vi "XXX_withREPLAN_PathPlanner_Cmd_Follow_Internal_Replan_Sample.vi"(4 "PassthroughTime_SEC":dbl, 5 "Extra Time Sec":dbl, 6 "Reset In":bool, 7 "ReplanningConfig":T6={"enableInitialReplanning"=TRUE, "enableDynamicReplanning"=FALSE, "dynamicReplanningTotalErrorThreshold"=1.0, "dynamicReplanningErrorSpikeThreshold"=0.25}, 8 "Position Error M":dbl, 9 "Current Pose SI":T20 {"ROTATION"."SIN" format="%13.4f"; "ROTATION"."COS" format="%13.4f"; "ROTATION"."VALUE" format="%13.4f"; "TRANSLATION"."Y" format="%14.3f"; "TRANSLATION"."X" format="%14.3f"}, 10 "CurrentChassisSpeeds":T21 {"vOmega" format="%10.3f"; "vY" format="%10.3f"; "vX" format="%10.3f"}, 11 "RePlannedPath in":T11={"Reversed"=FALSE, "RotationTargets"=[], "ConstraintZones"=[], "EventMarkers"=[], "GlobalConstraints"={"MaxVelocityMps;"=0.0, "MaxAccelerationMpsSq;"=0.0, "MaxAngularVelRadPsEc;"=0.0, "MaxAngularAccRadPSecSq"=0.0, "Exists"=FALSE, "Unlimited"=FALSE, "NominalVoltageVolts"=12.0}, "GoalEndState"={"VelocityMPS"=0.0, "Rotation"={"VALUE"=0.0, "COS"=0.0, "SIN"=0.0}}, "AllPoints"=[], "Name"="", "Waypoints"=[], "PointTowardsZones"=[], "IdealStartingState"={"VelocityMPS"=0.0, "Rotation"={"VALUE"=0.0, "COS"=0.0, "SIN"=0.0}}, "IsChoreoPath"=FALSE, "PreventFlipping"=FALSE} {"IdealStartingState"."Rotation"."SIN" format="%13.4f"; "IdealStartingState"."Rotation"."COS" format="%13.4f"; "IdealStartingState"."Rotation"."VALUE" format="%13.4f"; "PointTowardsZones"."TargetPosition"."Y" format="%14.3f"; "PointTowardsZones"."TargetPosition"."X" format="%14.3f"; "PointTowardsZones"."RotationOffset"."SIN" format="%13.4f"; "PointTowardsZones"."RotationOffset"."COS" format="%13.4f"; "PointTowardsZones"."RotationOffset"."VALUE" format="%13.4f"; "Waypoints"."nextControl"."Y" format="%14.3f"; "Waypoints"."nextControl"."X" format="%14.3f"; "Waypoints"."anchor"."Y" format="%14.3f"; "Waypoints"."anchor"."X" format="%14.3f"; "Waypoints"."prevControl"."Y" format="%14.3f"; "Waypoints"."prevControl"."X" format="%14.3f"; "AllPoints"."RotationTarget"."rotation"."SIN" format="%13.4f"; "AllPoints"."RotationTarget"."rotation"."COS" format="%13.4f"; "AllPoints"."RotationTarget"."rotation"."VALUE" format="%13.4f"; "AllPoints"."Position"."Y" format="%14.3f"; "AllPoints"."Position"."X" format="%14.3f"; "GoalEndState"."Rotation"."SIN" format="%13.4f"; "GoalEndState"."Rotation"."COS" format="%13.4f"; "GoalEndState"."Rotation"."VALUE" format="%13.4f"; "RotationTargets"."rotation"."SIN" format="%13.4f"; "RotationTargets"."rotation"."COS" format="%13.4f"; "RotationTargets"."rotation"."VALUE" format="%13.4f"}) -> (0 "Traj End Status":T5, 1 "Trajectory State":T7={"TimeSeconds"=0.0, "VelocityMPS"=0.0, "AccerationMpsSq"=0.0, "HeadingAngularVelRadPerSec"=0.0, "PositionMeters"={"X"=0.0, "Y"=0.0}, "Heading"={"VALUE"=0.0, "COS"=1.0, "SIN"=0.0}, "TargetHolonomicRotation"={"VALUE"=0.0, "COS"=1.0, "SIN"=0.0}, "CurvatureRadPerMeter"=0.0, "PathPlannerConstraints"={"MaxVelocityMps;"=0.0, "MaxAccelerationMpsSq;"=0.0, "MaxAngularVelRadPsEc;"=0.0, "MaxAngularAccRadPSecSq"=0.0, "Exists"=FALSE, "Unlimited"=FALSE, "NominalVoltageVolts"=12.0}, "DeltaPos"=0.0} {"TargetHolonomicRotation"."SIN" format="%13.4f"; "TargetHolonomicRotation"."COS" format="%13.4f"; "TargetHolonomicRotation"."VALUE" format="%13.4f"; "Heading"."SIN" format="%13.4f"; "Heading"."COS" format="%13.4f"; "Heading"."VALUE" format="%13.4f"; "PositionMeters"."Y" format="%14.3f"; "PositionMeters"."X" format="%14.3f"}, 2 "Reset Controller":bool, 3 "PathPlannerTrajectoryEvents":T1)   [LabVIEW 2019]
doc: "This is an internal function. It is not to be called by end users."
uses:
  <vilib>/Rock Robotics/WPI/ThirdParty/JAS_Junk/TrajLib/TypeDef/CHASSIS_SPEEDS.ctl
  <vilib>/Rock Robotics/WPI/ThirdParty/JAS_Junk/TrajLib/TypeDef/POSE2D.ctl
  <vilib>/Rock Robotics/WPI/ThirdParty/JAS_Junk/TrajLib/TypeDef/TRANSLATION2D.ctl
  <vilib>/Rock Robotics/WPI/ThirdParty/JAS_Junk/TrajLib/TypeDef/ROTATION2D.ctl
  PathPlannerLib24/TypeDef/PathPlannerPath.ctl
  PathPlannerLib24/TypeDef/PathPlannerRotationTarget.ctl
  PathPlannerLib24/TypeDef/PathPlannerConstraintsZone.ctl
  PathPlannerLib24/TypeDef/PathPlannerPathConstraints.ctl
  PathPlannerLib24/TypeDef/PathPlannerEventMarker.ctl
  PathPlannerLib24/TypeDef/PathPlannerCommandUtil.ctl
  PathPlannerLib24/ENum/PathPlanner_CommandUtilType_ENUM.ctl
  PathPlannerLib24/TypeDef/PathPlannerGoalEndState.ctl
  PathPlannerLib24/TypeDef/PathPlannerPathPoint.ctl
  PathPlannerLib24/TypeDef/PathPlannerWaypoint.ctl
  PathPlannerLib24/TypeDef/PathPlannerPointTowardsZone.ctl
  PathPlannerLib24/TypeDef/PathPlannerIdealStartingState.ctl
  PathPlannerLib24/TypeDef/PathPlannerTrajectoryState.ctl
  PathPlannerLib24/TypeDef/PathPlannerReplanningConfig.ctl
  PathPlannerLib24/TypeDef/PathPlannerTrajectoryEvents.ctl
  PathPlannerLib24/TypeDef/PathPlannerTrajectoryEvent.ctl
  <vilib>/Rock Robotics/WPI/ThirdParty/JAS_Junk/TrajLib/Rotation2d_GetDegrees.vi
  <vilib>/Rock Robotics/WPI/ThirdParty/JAS_Junk/TrajLib/MathUtil_InputModulus.vi
  <vilib>/Rock Robotics/WPI/ThirdParty/JAS_Junk/TrajLib/Rotation2d_CreateAngleDegrees.vi
  <vilib>/Rock Robotics/WPI/ThirdParty/JAS_Junk/TrajLib/Rotation2d_GetRadians.vi
  <vilib>/Rock Robotics/WPI/ThirdParty/JAS_Junk/TrajLib/Conv_Radians_Deg.vi
  <vilib>/Rock Robotics/WPI/ThirdParty/JAS_Junk/TrajLib/Conv_Deg_Radians.vi
  <vilib>/Rock Robotics/WPI/ThirdParty/JAS_Junk/TrajLib/Rotation2d_CreateAngle.vi
  <vilib>/Utility/semaphor.llb/Obtain Semaphore Reference.vi
  PathPlannerLib24/PathPlanner24.lvlib
  <vilib>/Rock Robotics/WPI/ThirdParty/JAS_Junk/TrajLib/Trajectory_Library.lvlib
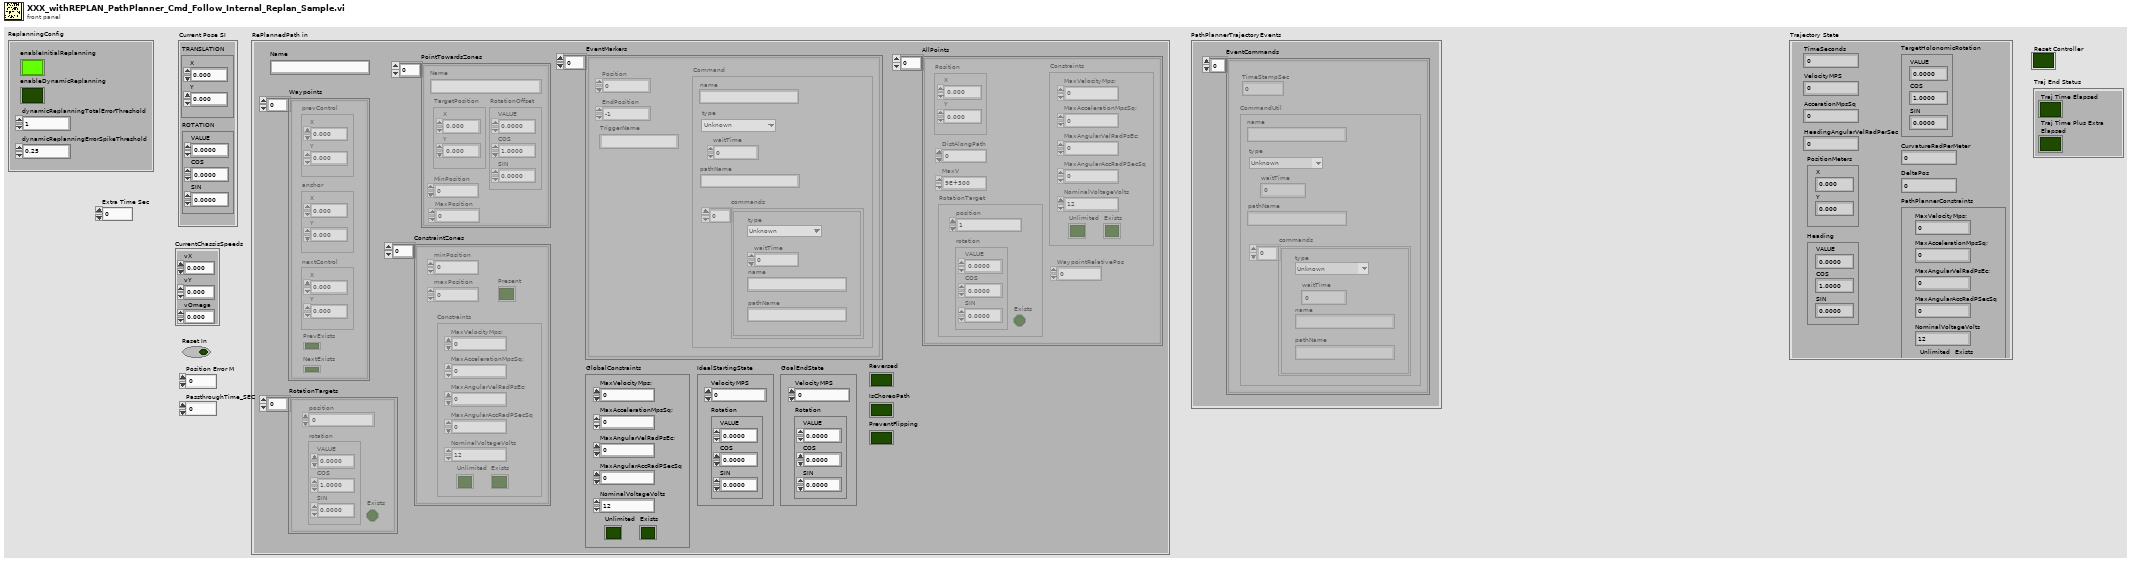
[diagram p1: front panel]
types:
  T1 = typedef "PathPlanner24.lvlib/PathPlannerTrajectoryEvents.ctl" = cluster{"EventCommands":T2[]}
  T2 = typedef "PathPlanner24.lvlib/PathPlannerTrajectoryEvent.ctl" = cluster{"TimeStampSec":dbl, "CommandUtil":T3}
  T3 = typedef "PathPlanner24.lvlib/PathPlannerCommandUtil.ctl" = cluster{"waitTime":dbl, "name":string, "pathName":string, "commands":cluster{"type":T4, "waitTime":dbl, "name":string, "pathName":string}[], "type":T4}
  T4 = typedef "PathPlanner24.lvlib/PathPlanner_CommandUtilType_ENUM.ctl" = enum16{"Unknown", "Wait", "Named", "Path", "Sequential", "Parallel", "Race", "Deadline"}
  T5 = cluster{"Traj Time Plus Extra\nElapsed":bool, "Traj Time Elapsed":bool}
  T6 = typedef "PathPlanner24.lvlib/PathPlannerReplanningConfig.ctl" = cluster{"enableInitialReplanning":bool, "enableDynamicReplanning":bool, "dynamicReplanningTotalErrorThreshold":dbl, "dynamicReplanningErrorSpikeThreshold":dbl}
  T7 = typedef "PathPlanner24.lvlib/PathPlannerTrajectoryState.ctl" = cluster{"TimeSeconds":dbl, "VelocityMPS":dbl, "AccerationMpsSq":dbl, "HeadingAngularVelRadPerSec":dbl, "PositionMeters":T8, "Heading":T9, "TargetHolonomicRotation":T9, "CurvatureRadPerMeter":dbl, "PathPlannerConstraints":T10, "DeltaPos":dbl}
  T8 = typedef "Trajectory_Library.lvlib/TRANSLATION2D.ctl" = cluster{"X":dbl, "Y":dbl}
  T9 = typedef "Trajectory_Library.lvlib/ROTATION2D.ctl" = cluster{"VALUE":dbl, "COS":dbl, "SIN":dbl}
  T10 = typedef "PathPlanner24.lvlib/PathPlannerPathConstraints.ctl" = cluster{"MaxVelocityMps;":dbl, "MaxAccelerationMpsSq;":dbl, "MaxAngularVelRadPsEc;":dbl, "MaxAngularAccRadPSecSq":dbl, "Exists":bool, "Unlimited":bool, "NominalVoltageVolts":dbl}
  T11 = typedef "PathPlanner24.lvlib/PathPlannerPath.ctl" = cluster{"Reversed":bool, "RotationTargets":T12[], "ConstraintZones":T13[], "EventMarkers":T14[], "GlobalConstraints":T10, "GoalEndState":T15, "AllPoints":T16[], "Name":string, "Waypoints":T17[], "PointTowardsZones":T18[], "IdealStartingState":T19, "IsChoreoPath":bool, "PreventFlipping":bool}
  T12 = typedef "PathPlanner24.lvlib/PathPlannerRotationTarget.ctl" = cluster{"position":dbl, "rotation":T9, "Exists":bool}
  T13 = typedef "PathPlanner24.lvlib/PathPlannerConstraintsZone.ctl" = cluster{"minPosition":dbl, "maxPosition":dbl, "Constraints":T10, "Present":bool}
  T14 = typedef "PathPlanner24.lvlib/PathPlannerEventMarker.ctl" = cluster{"Position":dbl, "Command":T3, "TriggerName":string, "EndPosition":dbl}
  T15 = typedef "PathPlanner24.lvlib/PathPlannerGoalEndState.ctl" = cluster{"VelocityMPS":dbl, "Rotation":T9}
  T16 = typedef "PathPlanner24.lvlib/PathPlannerPathPoint.ctl" = cluster{"Position":T8, "DistAlongPath":dbl, "MaxV":dbl, "Constraints":T10, "RotationTarget":T12, "WaypointRelativePos":dbl}
  T17 = typedef "PathPlanner24.lvlib/PathPlannerWaypoint.ctl" = cluster{"prevControl":T8, "anchor":T8, "nextControl":T8, "PrevExists":bool, "NextExists":bool}
  T18 = typedef "PathPlanner24.lvlib/PathPlannerPointTowardsZone.ctl" = cluster{"RotationOffset":T9, "Name":string, "TargetPosition":T8, "MinPosition":dbl, "MaxPosition":dbl}
  T19 = typedef "PathPlanner24.lvlib/PathPlannerIdealStartingState.ctl" = cluster{"VelocityMPS":dbl, "Rotation":T9}
  T20 = typedef "Trajectory_Library.lvlib/POSE2D.ctl" = cluster{"TRANSLATION":T8, "ROTATION":T9}
  T21 = typedef "Trajectory_Library.lvlib/CHASSIS_SPEEDS.ctl" = cluster{"vX":dbl, "vY":dbl, "vOmega":dbl}
  T22 = typedef "PathPlanner24.lvlib/PathPlannerTrajectory.ctl" = cluster{"States":T7[]}
  T23 = typedef "Trajectory_Library.lvlib/TIMER.ctl" = cluster{"StartTime":dbl, "Accumulated TIme":dbl, "Running":bool, "semaphore":T24}
  T24 = typedef "Semaphore RefNum" = refnum<k1>
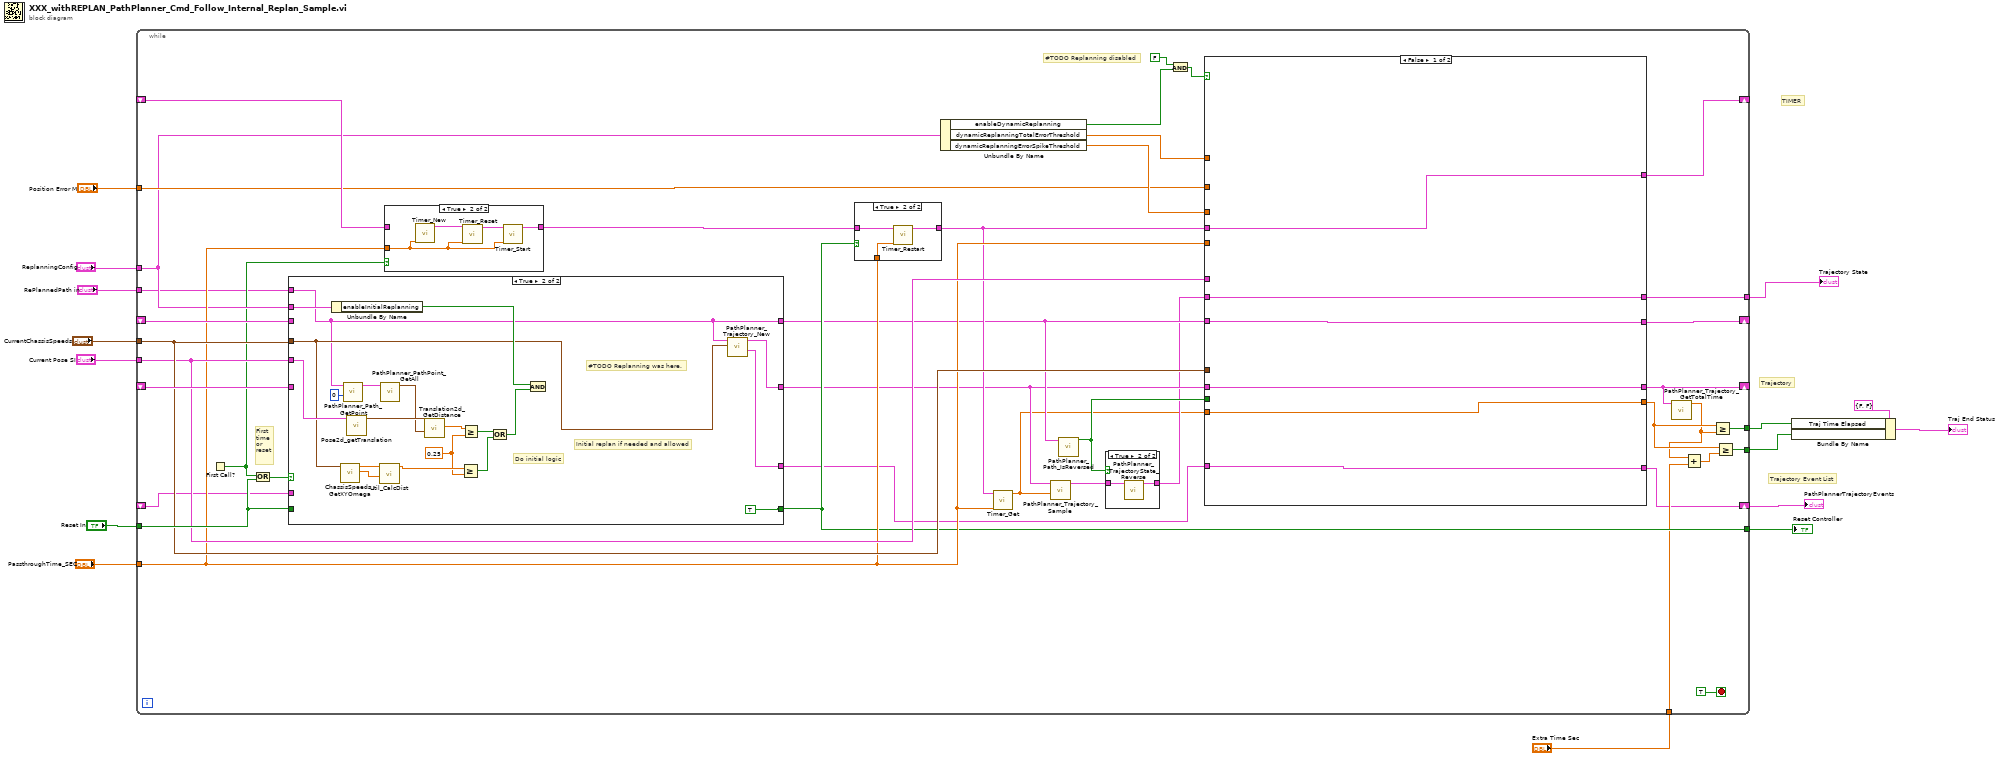
[diagram p0: block diagram]
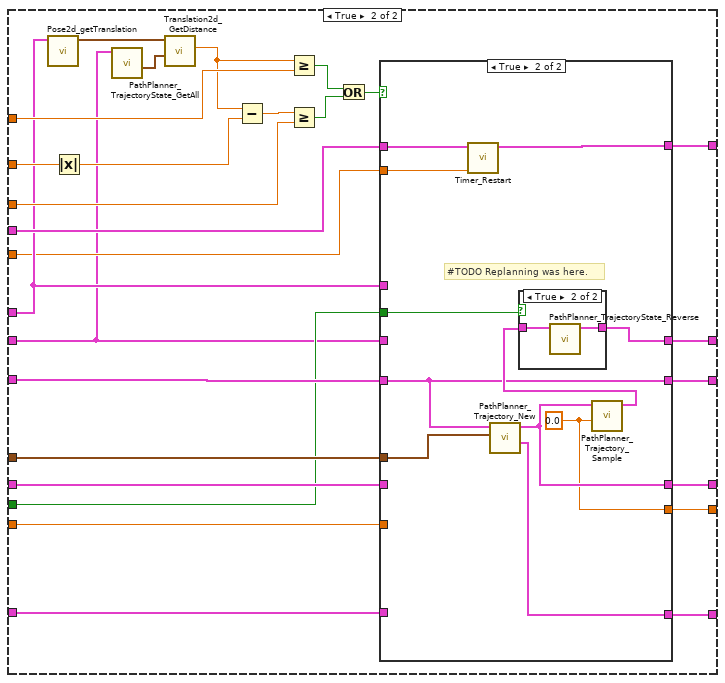
[diagram p2: hidden frame]
diagram:
  # "Trajectory Event List"
  # "TIMER"
  # "Trajectory"
  n1 = while {
    tunnel: "CurrentChassisSpeeds" -> [w50]
    tunnel: "Current Pose SI" -> [w49]
    shift-right: [w33] -> _
    shift-left: _ -> [w55]
    shift-right: [w40] -> _
    shift-left: _ -> [w54]
    tunnel: "Reset In" -> [w53]
    tunnel: [w39] -> w13
    tunnel: [w41] -> w11
    tunnel: "PassthroughTime_SEC" -> [w46]
    shift-right: [w35] -> _
    shift-left: _ -> [w47]
    tunnel: "Position Error M" -> [w38]
    tunnel: "ReplanningConfig" -> [w37]
    tunnel: [w32] -> w5
    tunnel: [w27] -> w4
    tunnel: "Extra Time Sec" -> [w26]
    shift-right: [w21] -> w1
    shift-left: _ -> [w20]
    tunnel: "RePlannedPath in" -> [w19]
    stop <- TRUE stop-if-true
    # "#TODO Replanning disabled"
    # "First\ntime\nor \nreset"
    n2 = First Call?() -> (First Call?: T/F=w34:bool)
    n3 = Or(x=w34, y=w53) -> (x .or. y?=w52:bool)
    n4 = case shown="True" w52 {
      tunnel: w54 -> [w123 _]
      tunnel: w50 -> [_ w129]
      tunnel: [w122 w128] -> w31
      tunnel: w37 -> [_ w143]
      tunnel: w49 -> [_ w130]
      tunnel: [w123 w127] -> w36
      tunnel: w55 -> [w122 _]
      tunnel: w53 -> [w124 _]
      tunnel: [w124 TRUE] -> w39
      tunnel: [w121 w125] -> w22
      tunnel: w20 -> [w121 _]
      tunnel: w19 -> [_ w127]
      frame False {
      }
      frame True {
        w132 = 0.25 ("y")
        # "#TODO Replanning was here."
        # "Initial replan if needed and allowed"
        # "Do initial logic"
        n5 = Unbundle By Name(w143) -> ("enableInitialReplanning"=w136:bool)
        n6 = call <vilib>:"ChassisSpeeds_GetXYOmega.vi"("CHASSIS"=w129) -> ("vY"=w134:dbl, "vX"=w135:dbl)  [unwired: 8 in, 1 out]
        n7 = call "PathPlanner_Path_GetPoint.vi"("Index"=0, "PathPlannerPath"=w127) -> ("Point"=w141:T16)  [unwired: 9 in]
        n8 = call <vilib>:"Pose2d_getTranslation.vi"("in POSE"=w130) -> ("outTRANSLATION"=w142:T8)  [unwired: 10 in]
        n9 = call <vilib>:"Util_CalcDist.vi"("Y"=w134, "X"=w135) -> ("DIST"=w133:dbl)  [unwired: 9 in]
        n10 = call "PathPlanner_PathPoint_GetAll.vi"("PathPlannerPoint"=w141) -> ("Position"=w140:T8)  [unwired: 5 in, 5 out]
        n11 = call <vilib>:"Translation2d_GetDistance.vi"("other Translation"=w140, "In Translation"=w142) -> ("Distance"=w139:dbl)  [unwired: 9 in]
        n12 = Greater Or Equal?(x=w133, y=w132) -> (x >= y?=w131:bool)
        n13 = Greater Or Equal?(x=w139, y=w132) -> (x >= y?=w138:bool)
        n14 = Or(x=w138, y=w131) -> (x .or. y?=w137:bool)
        n15 = And(x=w136, y=w137) -> ()  [unwired: 1 out]
        n16 = call "PathPlanner_Trajectory_New.vi"("StartingSpeeds"=w129, "Path"=w127) -> ("PathPlannerTrajectoryEvents"=w125:T1, "PathPlannerTrajectory"=w128:T22)  [unwired: 8 in]
      }
    }
    n17 = case shown="True" w34 {
      tunnel: w46 -> [_ w118]
      tunnel: [w116 w117] -> w48
      tunnel: w47 -> [w116 _]
      frame False {
      }
      frame True {
        n18 = call <vilib>:"Timer_New.vi"("Pass_Through_Time"=w118) -> ("TIMER"=w120:T23)  [unwired: 10 in]
        n19 = call <vilib>:"Timer_Reset.vi"("Pass_Through_Time"=w118, "in TIMER"=w120) -> ("out TIMER"=w119:T23)  [unwired: 9 in]
        n20 = call <vilib>:"Timer_Start.vi"("Pass_Through_Time"=w118, "in Timer"=w119) -> ("out Timer"=w117:T23)  [unwired: 9 in]
      }
    }
    n21 = case shown="True" w39 {
      tunnel: w48 -> [w109 w112]
      tunnel: [w109 w111] -> w43
      tunnel: w46 -> [_ w110]
      frame False {
      }
      frame True {
        n22 = call <vilib>:"Timer_Restart.vi"("Pass_Through_Time"=w110, "in Timer"=w112) -> ("out Timer"=w111:T23)  [unwired: 9 in]
      }
    }
    n23 = Unbundle By Name(w37) -> ("enableDynamicReplanning"=w17:bool, "dynamicReplanningTotalErrorThreshold"=w44:dbl, "dynamicReplanningErrorSpikeThreshold"=w45:dbl)
    n24 = call <vilib>:"Timer_Get.vi"("Pass_Through_Time"=w46, "TIMER"=w43) -> ("CurrentTImer"=w23:dbl)  [unwired: 9 in]
    n25 = call "PathPlanner_Trajectory_Sample.vi"("Time"=w23, "PathPlannerTrajectory"=w31) -> ("PathPlannerState"=w42:T7)  [unwired: 9 in]
    n26 = call "PathPlanner_Path_IsReversed.vi"("PathPlannerPath"=w36) -> ("Reversed"=w25:bool)  [unwired: 10 in]
    n27 = case shown="True" w25 {
      tunnel: w42 -> [w113 w115]
      tunnel: [w113 w114] -> w24
      frame False {
      }
      frame True {
        n28 = call "PathPlanner_TrajectoryState_Reverse.vi"("PathPlannerState"=w115) -> ("Reversed State"=w114:T7)  [unwired: 10 in]
      }
    }
    n29 = And(x=FALSE, y=w17) -> (x .and. y?=w18:bool)
    n30 = case shown="False" w18 {
      tunnel: w38 -> [_ w88]
      tunnel: w43 -> [w61 w79]
      tunnel: [w61 w78] -> w35
      tunnel: w49 -> [_ w75]
      tunnel: w44 -> [_ w85]
      tunnel: w45 -> [_ w81]
      tunnel: [w59 w77] -> w40
      tunnel: [w58 w76] -> w41
      tunnel: w50 -> [_ w74]
      tunnel: w31 -> [w60 w73]
      tunnel: [w60 w72] -> w33
      tunnel: w46 -> [_ w69]
      tunnel: w36 -> [w59 w68]
      tunnel: [w57 w67] -> w30
      tunnel: w25 -> [_ w66]
      tunnel: w24 -> [w58 w65]
      tunnel: w23 -> [w57 w64]
      tunnel: w22 -> [w56 w63]
      tunnel: [w56 w62] -> w21
      frame False {
      }
      frame True {
        n31 = call <vilib>:"Pose2d_getTranslation.vi"("in POSE"=w75) -> ("outTRANSLATION"=w86:T8)  [unwired: 10 in]
        n32 = Absolute Value(x=w88) -> (abs(x)=w84:dbl)
        n33 = call "PathPlanner_TrajectoryState_GetAll.vi"("PathPlannerState"=w65) -> ("PositionMeters"=w87:T8)  [unwired: 1 in, 9 out]
        n34 = call <vilib>:"Translation2d_GetDistance.vi"("other Translation"=w87, "In Translation"=w86) -> ("Distance"=w83:dbl)  [unwired: 9 in]
        n35 = Subtract(x=w83, y=w84) -> (x-y=w82:dbl)
        n36 = Greater Or Equal?(x=w83, y=w85) -> (x >= y?=w70:bool)
        n37 = Greater Or Equal?(x=w82, y=w81) -> (x >= y?=w71:bool)
        n38 = Or(x=w70, y=w71) -> (x .or. y?=w80:bool)
        n39 = case shown="True" w80 {
          tunnel: w79 -> [w94 w105]
          tunnel: [w94 w104] -> w78
          tunnel: w68 -> [w93 w95]
          tunnel: [w93 w95] -> w77
          tunnel: w65 -> [w92 _]
          tunnel: [w92 w100] -> w76
          tunnel: w75 -> [_ _]
          tunnel: w74 -> [_ w103]
          tunnel: w73 -> [w91 _]
          tunnel: [w91 w102] -> w72
          tunnel: w66 -> [_ w99]
          tunnel: w69 -> [_ w98]
          tunnel: [w90 w97] -> w67
          tunnel: w64 -> [w90 _]
          tunnel: w63 -> [w89 _]
          tunnel: [w89 w96] -> w62
          frame False {
          }
          frame True {
            w97 = 0.0 ("Time")
            # "#TODO Replanning was here."
            n40 = call <vilib>:"Timer_Restart.vi"("Pass_Through_Time"=w98, "in Timer"=w105) -> ("out Timer"=w104:T23)  [unwired: 9 in]
            n41 = call "PathPlanner_Trajectory_New.vi"("StartingSpeeds"=w103, "Path"=w95) -> ("PathPlannerTrajectoryEvents"=w96:T1, "PathPlannerTrajectory"=w102:T22)  [unwired: 8 in]
            n42 = call "PathPlanner_Trajectory_Sample.vi"("Time"=w97, "PathPlannerTrajectory"=w102) -> ("PathPlannerState"=w101:T7)  [unwired: 9 in]
            n43 = case shown="True" w99 {
              tunnel: w101 -> [w106 w108]
              tunnel: [w106 w107] -> w100
              frame False {
              }
              frame True {
                n44 = call "PathPlanner_TrajectoryState_Reverse.vi"("PathPlannerState"=w108) -> ("Reversed State"=w107:T7)  [unwired: 10 in]
              }
            }
          }
        }
      }
    }
    n45 = call "PathPlanner_Trajectory_GetTotalTime.vi"("PathPlannerTrajectory"=w33) -> ("TotalTimeSeconds"=w28:dbl)  [unwired: 10 in]
    n46 = Add(x=w28, y=w26) -> (x+y=w29:dbl)
    n47 = Greater Or Equal?(x=w30, y=w28) -> (x >= y?=w32:bool)
    n48 = Greater Or Equal?(x=w30, y=w29) -> (x >= y?=w27:bool)
  }
  "Reset Controller" <- w13
  "Trajectory State" <- w11
  "PathPlannerTrajectoryEvents" <- w1
  n49 = Bundle By Name(cluster=T5 {"Traj Time Plus Extra\nElapsed"=FALSE, "Traj Time Elapsed"=FALSE} ("Traj End Status"), "Traj Time Elapsed"=w5, "Traj Time Plus Extra\nElapsed"=w4) -> (→"Traj End Status":T5)
